vi "Read_Instr.vi"(8 "error in (no error)":errorcluster caption="entrée d'erreur (pas d'erreur)", 11 "Class Instrument Multimeter en entrée":refnum<class "Class Instrument Multimeter.lvclass">) -> (0 "error out":errorcluster caption="sortie d'erreur", 3 "Class Instrument Multimeter en sortie":refnum<class "Class Instrument Multimeter.lvclass">)   [LabVIEW 2020, in "Library Instrument & Equipement.lvlib" / "Library Instruments.lvlib" / "Class Instrument Multimeter.lvclass"]
uses:
  Class Instrument Multimeter.lvclass
  Class Instrument Multimeter.lvclass/Class Instrument Multimeter.ctl
  Instrument (Default)/Class Instrument (Default).lvclass
  Multimeter/Multimeter (Default)/Class Multimeter (Default).lvclass
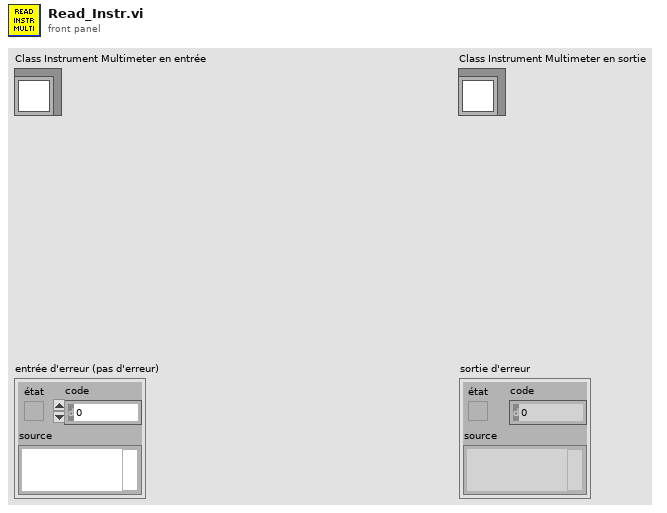
[diagram p1: front panel]
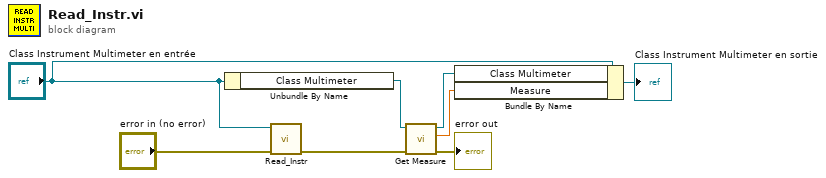
[diagram p0: block diagram]
diagram:
  n1 = Unbundle By Name("Class Instrument Multimeter en entrée") -> ("Class Multimeter"=w6:refnum<class "Class Multimeter (Default).lvclass">)
  n2 = call-parent "Read_Instr.vi"("error in (no error)"="error in (no error)", "Class Instrument (Default) en entrée"="Class Instrument Multimeter en entrée") -> ("error out"=w7:errorcluster)  [unwired: 8 in, 1 out]
  n3 = call-dynamic "Get Measure.vi"("error in (no error)"=w7, "Class Multimeter (Default) en entrée"=w6) -> ("error out"=→"error out":errorcluster, "Voltage"=w4:dbl, "Class Multimeter (Default) en sortie"=w1:refnum<class "Class Multimeter (Default).lvclass">)  [unwired: 7 in]
  n4 = Bundle By Name(cluster="Class Instrument Multimeter en entrée", "Class Multimeter"=w1, "Measure"=w4) -> (→"Class Instrument Multimeter en sortie":refnum<class "Class Instrument Multimeter.lvclass">)
